vi "事件结构.vi"() -> ()   [LabVIEW 2015]
panel:
  out "x*y":dbl
  in  "确定":bool
  out "布尔":bool
  in  "stop":bool
  in  "距离mm":u32 caption="Count(mSec)"
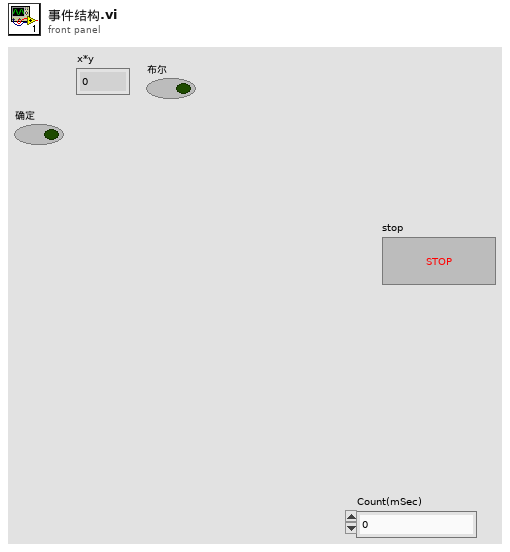
[diagram p1: front panel]
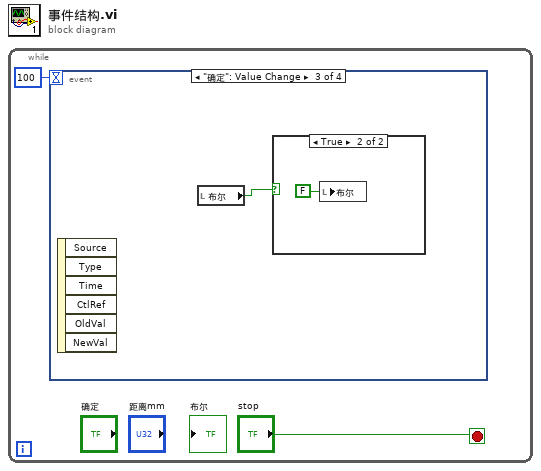
[diagram p0: block diagram]
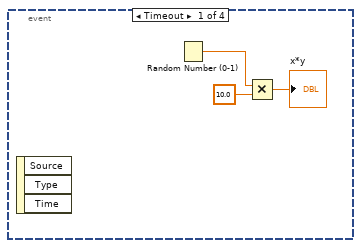
[diagram p2: hidden frame]
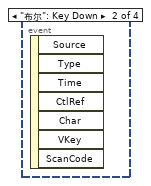
[diagram p3: hidden frame]
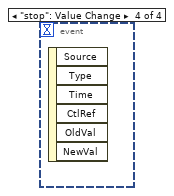
[diagram p5: hidden frame]
diagram:
  n1 = while {
    stop <- "stop" stop-if-true
    n2 = event shown="[2] \"确定\": Value Change" {
      selector: _ -> [_ _ _ _]
      dyn-events: _ -> [_ _ _ _]
      timeout: 100 -> [_ _ _ _]
      event Timeout {
        n3 = event-data() -> ()  [unwired: 1 in, 3 out]
        n4 = Random Number (0-1)() -> (number: 0 to 1=w5:dbl)
        n5 = Multiply(x=w5, y=10.0) -> (x*y=→"x*y":dbl)
      }
      event "布尔": Key Down {
        n6 = event-data() -> ()  [unwired: 1 in, 7 out]
      }
      event "确定": Value Change {
        n7 = event-data() -> ()  [unwired: 1 in, 6 out]
        n8 = local read "布尔"() -> (w6:bool)
        n9 = case shown="True" w6 {
          frame False {
          }
          frame True {
            n10 = local write "布尔"(FALSE ("布尔")) -> ()
          }
        }
      }
      event "stop": Value Change {
        n11 = event-data() -> ()  [unwired: 1 in, 6 out]
      }
    }
  }
